vi "Circular Path.vi"(11 "Trajectory Radius":dbl) -> (3 "Cluster":cluster{dbl[], dbl[]})   [LabVIEW 2021]
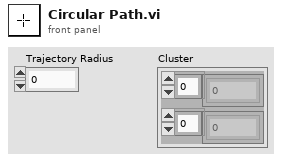
[diagram p1: front panel]
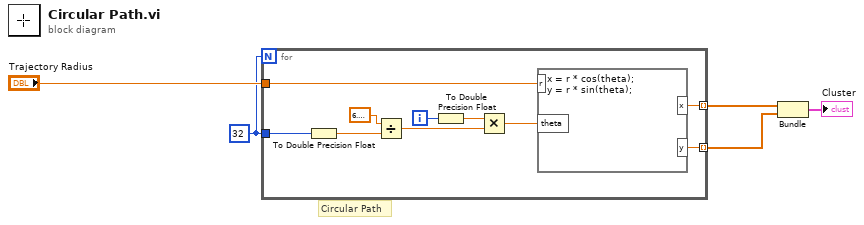
[diagram p0: block diagram]
diagram:
  w3 = 32 ("Drawing Samples")
  # "Circular Path"
  n1 = for {
    N: w3 -> [_]
    tunnel: [w15] -> w1 mode=indexing
    tunnel: [w14] -> w2 mode=indexing
    tunnel: w3 -> [w10]
    tunnel: "Trajectory Radius" -> [w6]
    i -> [w11]
    n2 = To Double Precision Float(number=w10) -> (double precision float=w8:dbl)
    n3 = Divide(x=6.283185307179586, y=w8) -> (x/y=w13:dbl)
    n4 = To Double Precision Float(number=w11) -> (double precision float=w9:dbl)
    n5 = Multiply(x=w9, y=w13) -> (x*y=w12:dbl)
    n6 = formula code="x = r * cos(theta);\ny = r * sin(theta);"("r"=w6, "theta"=w12) -> ("x"=w15:dbl, "y"=w14:dbl)
  }
  n7 = Bundle(w1, w2) -> (→"Cluster":cluster{dbl[], dbl[]})  [unwired: 1 in]
